vi "Pre Launch Init.vi"(11 "Mag Lab Hardware in":refnum<class "Mag Lab Hardware.lvclass">) -> (0 "error out":errorcluster, 3 "Mag Lab Hardware out":refnum<class "Mag Lab Hardware.lvclass">)   [LabVIEW 2015, in "Mag Lab Hardware.lvclass"]
doc: "(<B>Filename</B>: Actor Framework.lvlib:Actor.lvclass:Pre Launch Init.vi)\n\nDefines behavior that occurs after the Launch Actor method is invoked but before the actor's Actor Core method begins running.\n\nThe Pre Launch Init method is guaranteed to finish before the Launch Actor method returns to its caller and before the actor itself receives any messages. Any references that the Pre Launch Init method obtains are guaranteed to have the same lifetime as the actor itself. Any errors that the Pre Launch Init method returns will abort the launch.\n\nBy default, this method does nothing. A descendant class may override it to define behavior."
uses:
  Mag Lab Hardware.lvclass
  <vilib>/ActorFramework/Actor/Actor.lvclass/Actor.ctl
  Mag Lab Hardware.lvclass/Mag Lab Hardware.ctl
  Mag Lab Measure Base/Mag Lab Measure Base.lvclass
  <vilib>/ActorFramework/Actor/Actor.lvclass
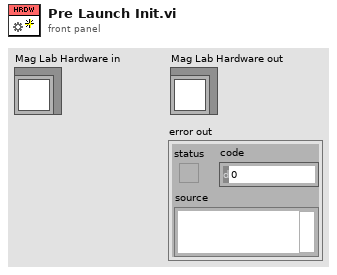
[diagram p1: front panel]
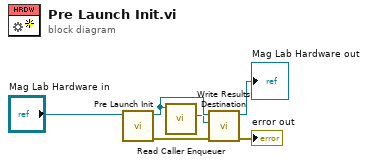
[diagram p0: block diagram]
diagram:
  n1 = call-parent "Pre Launch Init.vi"("Mag Lab Measure Base in"="Mag Lab Hardware in") -> ("error out"=w2:errorcluster, "Mag Lab Measure Base out"=w4:refnum<class "Mag Lab Hardware.lvclass">)  [unwired: 9 in]
  n2 = call <vilib>:"Read Caller Enqueuer.vi"("Actor"=w4) -> ("Caller Enqueuer"=w3:refnum<class "Message Enqueuer.lvclass">)  [unwired: 10 in]
  n3 = call "Write Results Destination.vi"("error in (no error)"=w2, "Actor Framework:Message Enqueuer"=w3, "Mag Lab Hardware in"=w4) -> ("error out"=→"error out":errorcluster, "Mag Lab Hardware out"=→"Mag Lab Hardware out":refnum<class "Mag Lab Hardware.lvclass">)  [unwired: 7 in]
